vi "Client Read Bytes Test.vi"() -> ()   [LabVIEW 2014, in "ESP8266 WiFi Wrapper.lvlib"]
uses:
  <vilib>/Aledyne-TSXperts/Arduino Compatible Compiler for LabVIEW/addons/ESP8266 WiFi Wrapper/ESP8266 WiFi Wrapper.lvlib
panel:
  out "Bytes read":i16
  out "Error Out":errorcluster
  in  "Error In":errorcluster
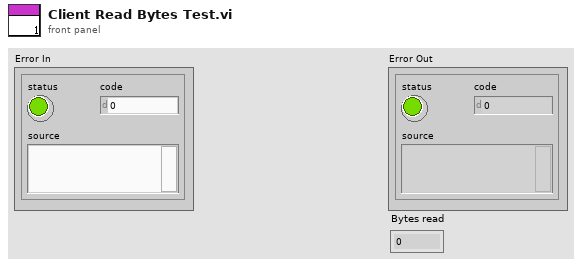
[diagram p1: front panel]
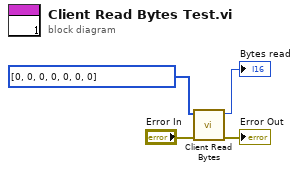
[diagram p0: block diagram]
diagram:
  n1 = call <vilib>:"Client Read Bytes.vi"("Error In"="Error In", "Buffer"=u8[] [0, 0, 0, 0, 0, 0, 0]) -> ("Error Out"=→"Error Out":errorcluster, "Bytes read"=→"Bytes read":i16)  [unwired: 8 in]
